vi "Add Notes to SR.vi"(8 "Error In":errorcluster, 9 "SR Number":i32, 10 "Note to Add":string, 11 "UI":refnum<queue>) -> (0 "Error Out":errorcluster)   [LabVIEW 2018]
uses:
  Support/Message Queue/Message Cluster.ctl
  Type Defs/FGV States.ctl
  Support/Message Queue/Enqueue Message (Single).vi
  Support/Message Queue/Message Queue.lvlib
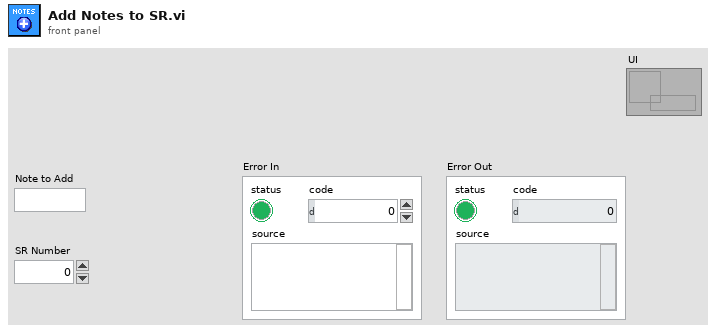
[diagram p1: front panel]
types:
  T1 = typedef "FGV States.ctl" = enum16{"Initialize", "Merge", "Write", "Remove", "Read", "Clear"}
  T2 = typedef "SR Cluster.ctl" = cluster{"Color":u32, "SR Number":i32, "SR Status":T3, "Name":string, "Summary":string, "Last Updated":timestamp, "SR Type":string, "Service Level":string, "Days Open":dbl, "Creation Date":timestamp, "Owner":string, "Note":string}
  T3 = typedef "SR Status.ctl" = enum16{"Caller Abandoned", "Created in Error", "Expired", "Forum Resolved AE", "Forum Resolved Customer", "IN WORK", "IN WORK Collab with AES", "IN WORK Collab with PSE", "IN WORK Collab with SE", "IN WORK Customer Added Note", "IN WORK Escalation", "IN WORK Wait on Customer", "Open", "Potentially Resolved", "Presumed Resolved", "RMA Approved for Return", "RMA Closed", "RMA Closed - DOA", "RMA In Progress", "RMA Open", "RMA Waiting on Customer", "Resolved", "Passed Off"}
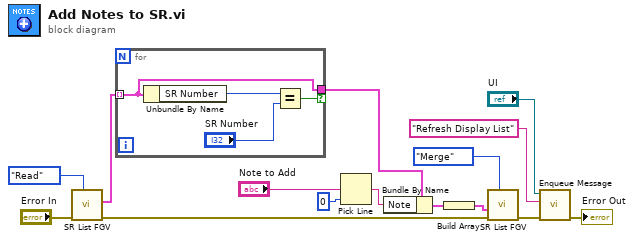
[diagram p0: block diagram]
diagram:
  n1 = call "SR List FGV.vi"("Operation"=FGV_States."Read", "Error In"="Error In") -> ("Error Out"=w4:errorcluster, "list out"=w11:T2[])  [unwired: 8 in]
  n2 = for {
    tunnel: w11 -> [w19] mode=indexing
    tunnel: [w19] -> w9 if=w18
    n3 = Unbundle By Name(w19) -> ("SR Number"=w16:i32)
    n4 = Equal?(x=w16, y="SR Number") -> (x = y?=w18:bool)
  }
  n5 = Pick Line(multi-line string="Note to Add", line index=0) -> (output string=w2:string)  [unwired: 1 in]
  n6 = Bundle By Name(cluster=w9, "Note"=w2) -> (w6:T2)
  n7 = Build Array(w6) -> (w5:T2[])
  n8 = call "SR List FGV.vi"("Operation"=FGV_States."Merge", "Error In"=w4, "Input"=w5) -> ("Error Out"=w7:errorcluster)  [unwired: 7 in, 1 out]
  n9 = call-poly "Enqueue Message.vi"("error in (no error)"=w7, "Message"="Refresh Display List", "Message Queue"="UI") -> ("error out"=→"Error Out":errorcluster)  [unwired: 7 in, 1 out]
